vi "Quadricoptère.vi"() -> ()   [LabVIEW 2011]
uses:
  Etats.ctl
  <vilib>/Instr/_visa.llb/VISA Configure Serial Port (Instr).vi
panel:
  in  "Onglets1":T1(tab)
  in  "stop":bool
  in  "connect":bool
  in  "Selection du port COM":refnum<visa-resource-name>="COM1"
  in  "disconnect":bool
  in  "Onglets2":T2(tab)
  out "Accéléromètre":T3(graph)
  out "Gyroscope":T3(graph)
  out "AnglesGyro":T3(graph)
  out "Pression":T3(graph)
  out "Température":T3(graph)
  out "Magnétomètre":T3(graph)
  out "Altitude":T3(graph)
  out "Tension":T3(graph)
  out "Courant":T3(graph)
  out "PWM":T3(graph)
  in  "Onglets3":enum32{"Moteurs", "Gains"}(tab)
  in  "Moteur 4":dbl(knob) min=0.0 max=100.0 step=1.0 scale=0.0..100.0 scale format="%#.2g"
  in  "Moteur 3":dbl(knob) min=0.0 max=100.0 step=1.0 scale=0.0..100.0 scale format="%#.2g"
  in  "Moteur 2":dbl(knob) min=0.0 max=100.0 step=1.0 scale=0.0..100.0 scale format="%#.2g"
  in  "Arreter moteurs":bool
  in  "Valider moteurs":bool
  in  "Moteur 1":dbl(knob) min=0.0 max=100.0 step=1.0 scale=0.0..100.0 scale format="%#.2g"
  out "Log RS232":string
  out "Etat":T4
  out "Dernière Commande":string
  out "File d'attente":i32
  # "Pas fonctionnel !"
  # "Pas fonctionnel !"
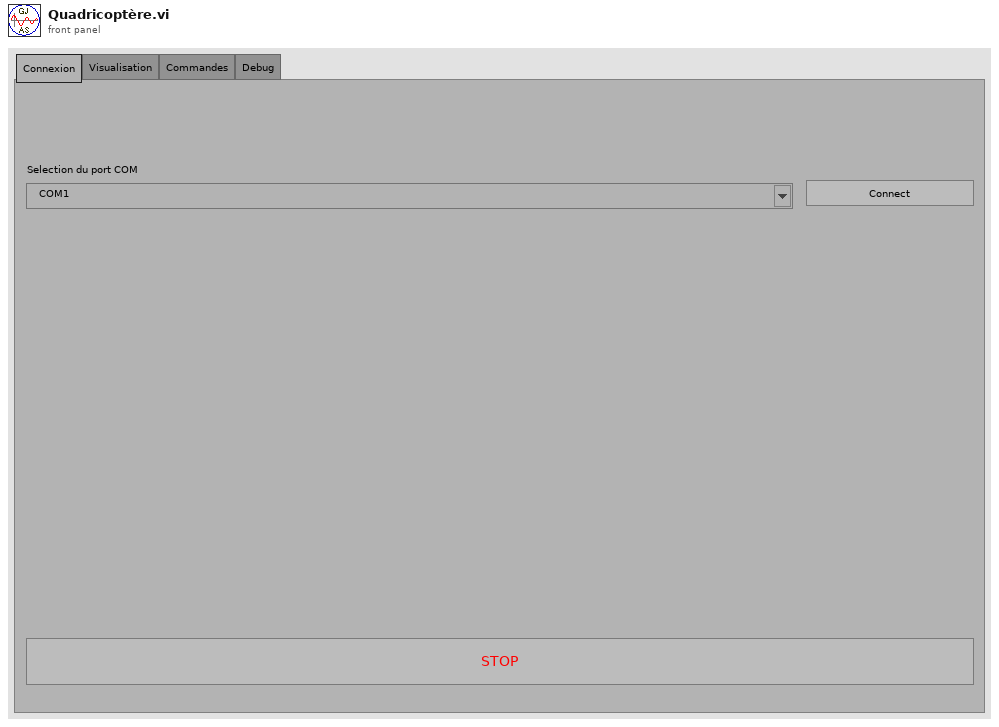
[diagram p1: front panel]
types:
  T1 = enum32{"Connexion", "Visualisation", "Commandes", "Debug"}
  T2 = enum32{"Accéléromètre", "Gyroscope", "Angles gyroscope", "Pression", "Température", "Magnétomètre", "Altitude", "Tension accu", "Courant accu", "Signaux PWM"}
  T3 = cluster{"Val 1":dbl, "Val 2":dbl, "Val 3":dbl, "Val 4":dbl, "Val 5":dbl}
  T4 = typedef "Etats.ctl" = enum16{"Init", "Wait", "Connect", "Read", "Process", "Test commandes", "Set Moteurs", "Reset Moteurs", "Disconnect"}
  T5 = typedef "Capteurs.ctl" = enum16{"Commande invalide !", "Capteur invalide !", "Accéléromètre", "Gyroscope", "Pression", "Température", "Magnétomètre", "Altitude", "Tension accu", "Courant accu", "Angles gyroscope", "Duty cycle PWM"}
  T6 = enum8{"Enabled", "Disabled", "Disabled and Grayed Out"}
  T7 = enum32{"Page Enabled", "Page Disabled", "Page Disabled & Grayed"}
  T8 = cluster{"Val 1":dbl, "Val 2":dbl, "Val 3":dbl, "Val 4":dbl, "Val 5":dbl}[]
  T9 = cluster{"Pages[0]":refnum<vi>, "Pages[1]":refnum<vi>, "Pages[2]":refnum<vi>, "Pages[3]":refnum<vi>, "Pages[4]":refnum<vi>, "Pages[5]":refnum<vi>, "Pages[6]":refnum<vi>, "Pages[7]":refnum<vi>, "Pages[8]":refnum<vi>}
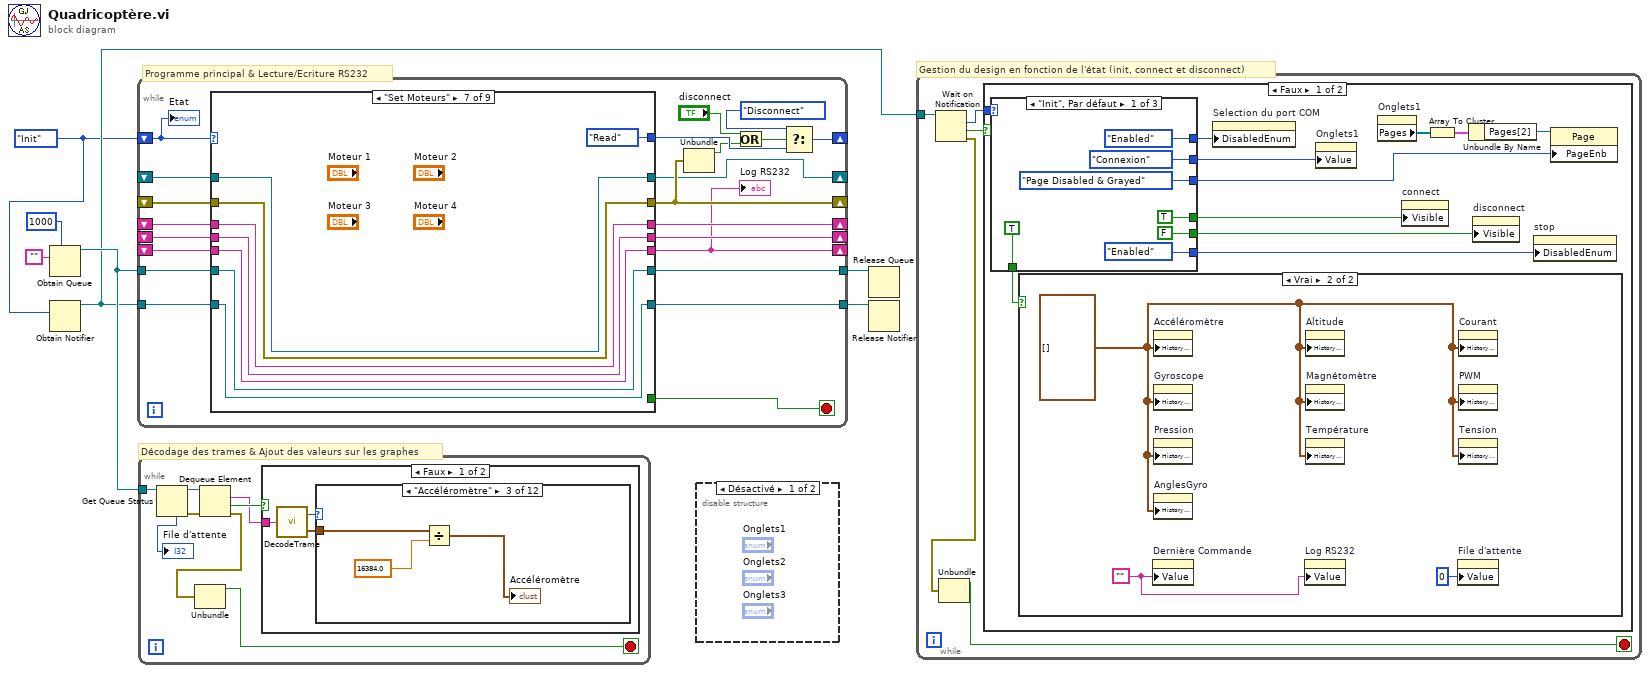
[diagram p0: block diagram]
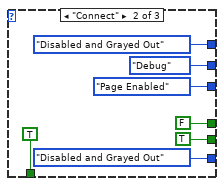
[diagram p3: hidden frame]
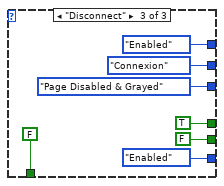
[diagram p4: hidden frame]
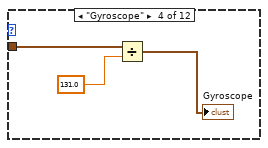
[diagram p9: hidden frame]
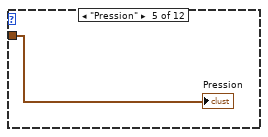
[diagram p10: hidden frame]
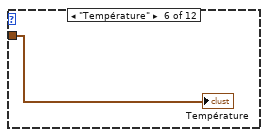
[diagram p11: hidden frame]
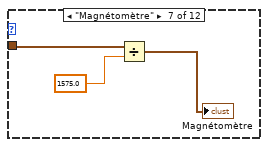
[diagram p12: hidden frame]
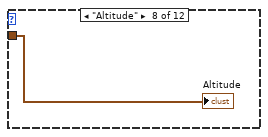
[diagram p13: hidden frame]
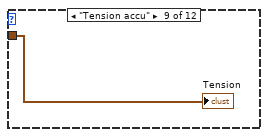
[diagram p14: hidden frame]
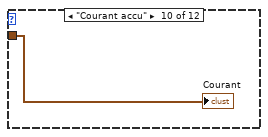
[diagram p15: hidden frame]
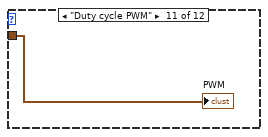
[diagram p16: hidden frame]
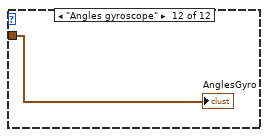
[diagram p17: hidden frame]
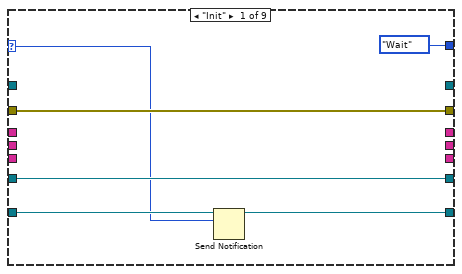
[diagram p19: hidden frame]
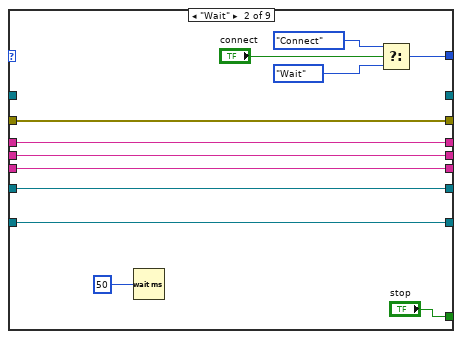
[diagram p20: hidden frame]
diagram:
  w2 = Etats."Init"
  # "Programme principal & Lecture/Ecriture RS232"
  # "Décodage des trames & Ajout des valeurs sur les graphes"
  # "Gestion du design en fonction de l'état (init, connect et disconnect)"
  n1 = Obtain Queue(max queue size (-1, unlimited)=1000 ("taille max de la file d'attente (-1, non limitée)"), element data type="") -> (queue out=w5:refnum<queue>)  [unwired: 3 in, 2 out]
  n2 = Obtain Notifier(notification data type=w2) -> (notifier out=w4:refnum<notifier>)  [unwired: 3 in, 2 out]
  n3 = while {
    shift-right: [w28] -> _
    shift-left: w2 -> [w10]
    shift-right: [w11] -> _
    shift-left: _ -> [w25]
    shift-right: [w23] -> _
    shift-left: _ -> [w26]
    shift-right: [w12] -> _
    shift-left: _ -> [w24]
    shift-right: [w21] -> _
    shift-left: _ -> [w22]
    shift-right: [w20] -> _
    shift-left: _ -> [w19]
    tunnel: [w15] -> w6
    tunnel: w5 -> [w14]
    tunnel: w4 -> [w8]
    tunnel: [w9] -> w3
    stop <- w13 stop-if-true
    n4 = case shown="\"Set Moteurs\"" w10 {
      selector: w10 -> [w30 _ w48 _ _ _ _ _ w115]
      tunnel: [Etats."Wait" w45 Etats."Read" w63 Etats."Test commandes" w87 Etats."Read" Etats."Read" Etats."Wait"] -> w29
      tunnel: [_ _ w56 w73 w75 w90 w99 w107 _] -> w11
      tunnel: [w33 w44 w55 w72 w79 w91 w100 w108 w120] -> w23
      tunnel: w26 -> [w33 w44 w53 w69 w80 w91 w100 w108 w126]
      tunnel: w25 -> [_ _ _ w70 w75 w90 w99 w107 w125]
      tunnel: [_ w42 _ w68 w83 w94 w103 w111 w124] -> w12
      tunnel: w24 -> [_ w42 _ w71 w83 w94 w103 w111 w124]
      tunnel: w22 -> [_ w40 _ w65 w81 w92 w101 w109 w119]
      tunnel: [_ w40 _ w64 w81 w92 w101 w109 w119] -> w21
      tunnel: [_ w39 _ w59 w78 w93 w102 w110 w118] -> w20
      tunnel: w19 -> [_ w39 _ _ w78 w93 w102 w110 w118]
      tunnel: [w34 w38 w51 w58 w76 w95 w104 w112 w117] -> w15
      tunnel: w14 -> [w34 w38 w51 w58 w77 w95 w104 w112 w117]
      tunnel: [_ "stop" _ _ _ _ _ _ _] -> w13
      tunnel: [w31 w36 w49 w57 w74 w96 w105 w113 w114] -> w9
      tunnel: w8 -> [w32 w36 w50 w57 w74 w96 w105 w113 w116]
      frame "Init" {
        n5 = Send Notification(notification=w30, notifier=w32) -> (notifier out=w31:refnum<notifier>)  [unwired: 1 in, 1 out]
      }
      frame "Wait" {
        n6 = Wait (ms)(milliseconds to wait=u32 50 ("attente (ms)")) -> ()  [unwired: 1 out]
        n7 = Select(t=Etats."Connect", s="connect", f=Etats."Wait") -> (s? t:f=w45:T4)
      }
      frame "Connect" {
        n8 = Send Notification(notification=w48, notifier=w50) -> (notifier out=w49:refnum<notifier>)  [unwired: 1 in, 1 out]
        n9 = call-poly "VISA Configure Serial Port"("VISA resource name"="Selection du port COM", "error in (no error)"=w53) -> ("VISA resource name out"=w56:refnum<visa-resource-name>, "error out"=w55:errorcluster)  [unwired: 12 in]
      }
      frame "Read" {
        n10 = call "ReceptionRS232.vi"("VISA in"=w70, "Erreur in"=w69) -> ("VISA out"=w73:refnum<visa-resource-name>, "Réponse"=w66:string, "Erreur out"=w72:errorcluster)
        n11 = Concatenate Strings(w65, w66) -> (w67:string)
        n12 = call "SplitTrame.vi"("Données IN"=w67) -> ("Données OUT"=w64:string, "Nouvelle commande"=w62:bool, "Commande"=w59:string)
        n13 = Concatenate Strings(w71, w66) -> (w68:string)
        n14 = Select(t=Etats."Process", s=w62, f=Etats."Test commandes") -> (s? t:f=w63:T4)
      }
      frame "Process" {
        n15 = Enqueue Element(queue=w77, element=w78, error in (no error)=w80) -> (queue out=w76:refnum<queue>, error out=w79:errorcluster)  [unwired: 1 in, 1 out]
        "Dernière Commande" <- w78
      }
      frame "Test commandes" {
        n16 = Select(t=Etats."Set Moteurs", s="Valider moteurs", f=Etats."Read") -> (s? t:f=w88:T4)
        n17 = Select(t=Etats."Reset Moteurs", s="Arreter moteurs", f=w88) -> (s? t:f=w87:T4)
      }
      frame "Set Moteurs" {
      }
      frame "Reset Moteurs" {
      }
      frame "Disconnect" {
        n18 = VISA Close(VISA resource name=w125, error in (no error)=w126) -> (error out=w122:errorcluster)
        n19 = call <vilib>:"Simple Error Handler.vi"("error in (no error)"=w122) -> ("error out"=w121:errorcluster)  [unwired: 4 in, 4 out]
        n20 = Send Notification(notification=w115, notifier=w116) -> (notifier out=w114:refnum<notifier>)  [unwired: 1 in, 1 out]
        n21 = call <vilib>:"Clear Errors.vi"("error in (no error)"=w121) -> ("error out"=w120:errorcluster)  [unwired: 6 in]
      }
    }
    "Log RS232" <- w12
    n22 = Unbundle(w23) -> ("status"=w18:bool)  [unwired: 2 out]
    n23 = Or(x="disconnect", y=w18) -> (x .or. y?=w16:bool)
    n24 = Select(t=Etats."Disconnect", s=w16, f=w29) -> (s? t:f=w28:T4)
    "Etat" <- w10
  }
  n25 = while {
    tunnel: w5 -> [w133]
    stop <- w127 stop-if-true
    n26 = Get Queue Status(queue=w133) -> (queue out=w132:refnum<queue>, error out=w129:errorcluster, # elements in queue=→"File d'attente":i32)  [unwired: 2 in, 5 out]
    n27 = Dequeue Element(queue=w132, error in (no error)=w129) -> (element=w130:string, timed out?=w131:bool, error out=w128:errorcluster)  [unwired: 1 in, 1 out]
    n28 = Unbundle(w128) -> ("status"=w127:bool)  [unwired: 2 out]
    n29 = case shown="Faux" w131 {
      tunnel: w130 -> [w135 _]
      frame False {
        n30 = call "DecodeTrame.vi"("Commande"=w135) -> ("Capteur"=w137:T5, "Valeurs"=w136:T3)
        n31 = case shown="\"Accéléromètre\"" w137 {
          tunnel: w136 -> [_ _ w140 w143 w144 w145 w148 w149 w150 w151 w152 w153]
          frame "Commande invalide !" {
          }
          frame "Capteur invalide !" {
          }
          frame "Accéléromètre" {
            n32 = Divide(x=w140, y=16384.0) -> (x/y=→"Accéléromètre":T3)
          }
          frame "Gyroscope" {
            n33 = Divide(x=w143, y=131.0) -> (x/y=→"Gyroscope":T3)
          }
          frame "Pression" {
            "Pression" <- w144
          }
          frame "Température" {
            "Température" <- w145
          }
          frame "Magnétomètre" {
            n34 = Divide(x=w148, y=1575.0) -> (x/y=→"Magnétomètre":T3)
          }
          frame "Altitude" {
            "Altitude" <- w149
          }
          frame "Tension accu" {
            "Tension" <- w150
          }
          frame "Courant accu" {
            "Courant" <- w151
          }
          frame "Duty cycle PWM" {
            "PWM" <- w152
          }
          frame "Angles gyroscope" {
            "AnglesGyro" <- w153
          }
        }
      }
      frame True {
      }
    }
  }
  n35 = disable-structure shown="Désactivé" {
    frame Disabled {
    }
    frame Enabled {
    }
  }
  n36 = Release Queue(queue=w6) -> ()  [unwired: 2 in, 3 out]
  n37 = Release Notifier(notifier=w3) -> ()  [unwired: 2 in, 3 out]
  n38 = while {
    tunnel: w4 -> [w157]
    stop <- w154 stop-if-true
    n39 = Wait on Notification(notifier=w157) -> (notification=w156:T4, timed out?=w158:bool, error out=w155:errorcluster)  [unwired: 3 in, 1 out]
    n40 = Unbundle(w155) -> ("status"=w154:bool)  [unwired: 2 out]
    n41 = case shown="Faux" w158 {
      tunnel: w156 -> [w169 _]
      frame False {
        n42 = case shown="\"Init\", Par défaut" w169 {
          tunnel: [T6."Enabled" ("Désactivé") T6."Disabled and Grayed Out" ("Désactivé") T6."Enabled" ("Désactivé")] -> w168
          tunnel: [T1."Connexion" ("Onglets1") T1."Debug" ("Onglets1") T1."Connexion" ("Onglets1")] -> w167
          tunnel: [TRUE ("Visible") FALSE ("Visible") TRUE ("Visible")] -> w166
          tunnel: [FALSE ("Visible") TRUE ("Visible") FALSE ("Visible")] -> w165
          tunnel: [T7."Page Disabled & Grayed" ("État d'activation de la page") T7."Page Enabled" ("État d'activation de la page") T7."Page Disabled & Grayed" ("État d'activation de la page")] -> w161
          tunnel: [TRUE ("Visible") TRUE ("Visible") FALSE ("Visible")] -> w160
          tunnel: [T6."Enabled" ("Désactivé") T6."Disabled and Grayed Out" ("Désactivé") T6."Enabled" ("Désactivé")] -> w159
          frame "Init", Default {
          }
          frame "Connect" {
          }
          frame "Disconnect" {
          }
        }
        n43 = case shown="Vrai" w160 {
          frame False {
          }
          frame True {
            w172 = ""
            w170 = T8 [] ("Données d'historique")
            n44 = property on="Dernière Commande" class="Ch"("Value"=w172) -> ()  [unwired: 2 in, 2 out]
            n45 = property on="Accéléromètre" class="GraphDér (strict)"("History Data"=w170) -> ()  [unwired: 2 in, 2 out]
            n46 = property on="Gyroscope" class="GraphDér (strict)"("History Data"=w170) -> ()  [unwired: 2 in, 2 out]
            n47 = property on="Pression" class="GraphDér (strict)"("History Data"=w170) -> ()  [unwired: 2 in, 2 out]
            n48 = property on="AnglesGyro" class="GraphDér (strict)"("History Data"=w170) -> ()  [unwired: 2 in, 2 out]
            n49 = property on="Log RS232" class="Ch"("Value"=w172) -> ()  [unwired: 2 in, 2 out]
            n50 = property on="Altitude" class="GraphDér (strict)"("History Data"=w170) -> ()  [unwired: 2 in, 2 out]
            n51 = property on="Magnétomètre" class="GraphDér (strict)"("History Data"=w170) -> ()  [unwired: 2 in, 2 out]
            n52 = property on="Température" class="GraphDér (strict)"("History Data"=w170) -> ()  [unwired: 2 in, 2 out]
            n53 = property on="File d'attente" class="NumNb (strict)"("Value"=0 ("File d'attente")) -> ()  [unwired: 2 in, 2 out]
            n54 = property on="Courant" class="GraphDér (strict)"("History Data"=w170) -> ()  [unwired: 2 in, 2 out]
            n55 = property on="PWM" class="GraphDér (strict)"("History Data"=w170) -> ()  [unwired: 2 in, 2 out]
            n56 = property on="Tension" class="GraphDér (strict)"("History Data"=w170) -> ()  [unwired: 2 in, 2 out]
          }
        }
        n57 = property on="Selection du port COM" class="NomVISA"("DisabledEnum"=w168) -> ()  [unwired: 2 in, 2 out]
        n58 = property on="Onglets1" class="Onglet (strict)"("Value"=w167) -> ()  [unwired: 2 in, 2 out]
        n59 = property on="Onglets1" class="Onglet (strict)"() -> ("Pages"=w163:refnum<vi>[])  [unwired: 2 in, 2 out]
        n60 = property on="connect" class="Bool"("Visible"=w166) -> ()  [unwired: 2 in, 2 out]
        n61 = Array To Cluster(array=w163) -> (cluster=w164:T9)
        n62 = Unbundle By Name(w164) -> ("Pages[2]"=w162:refnum<vi>)
        n63 = property on="disconnect" class="Bool"("Visible"=w165) -> ()  [unwired: 2 in, 2 out]
        n64 = property on="stop" class="Bool (strict)"("DisabledEnum"=w159) -> ()  [unwired: 2 in, 2 out]
        n65 = property class="Page"(reference=w162, "PageEnb"=w161) -> ()  [unwired: 1 in, 2 out]
      }
      frame True {
      }
    }
  }
